vi "VMR Server URL Const.vi"() -> (2 "VMR Server URL":string="192.168.42.50")   [LabVIEW 2022 SP3, in "TouchControl.lvlib"]
uses:
  TouchControl.lvlib
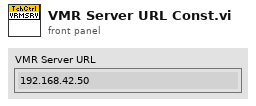
[diagram p1: front panel]
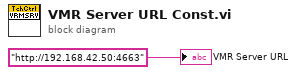
[diagram p0: block diagram]
diagram:
  "VMR Server URL" <- "http://192.168.42.50:4663"
